vi "Dashboard Main.vi"() -> ()   [LabVIEW 2013]
uses:
  <vilib>/event_ctls.llb/eventvkey.ctl
  <vilib>/Rock Robotics/WPI/Dashboard/WPI_DashboardLogging Global.vi
  <vilib>/Utility/config.llb/Write Key (String).vi
  <vilib>/Utility/config.llb/Write Key (I32).vi
  <vilib>/Utility/config.llb/NI_LVConfig.lvlib
panel:
  out "Image Message":string="Timeout in Camera Communications"
  in  "Rec Mode":enum32{"Stop", "Record", "Playback"}(radio)
  in  "Dashboard Tab":T1(tab)
  out "Maybe\nShoot?":bool
  out "DISTANCE":dbl
  in  "Camera Settings":T2={"Frame Rate"=30, "Compression"=30, "Size"=1} {"Frame Rate" scale=1.0..30.0; "Size" items=["640x480", "320x240", "160x120"]}
  out "MotorSliders R":cluster{"MotorSlide1":dbl, "MotorSlide2":dbl} {"MotorSlide2" scale=-1.0..1.0 scale format="%#_2e"; "MotorSlide1" scale=-1.0..1.0 scale format="%#_2e"}
  out "MotorChart R":cluster{"Numeric":dbl, "Numeric":dbl}(graph)
  out "MotorSliders L":T3 {"MotorSlide4 2" scale=0.0..14.0 scale format="%#_2e"; "MotorSlide2" scale=-1.0..1.0 scale format="%#_2e"; "MotorSlide1" scale=-1.0..1.0 scale format="%#_2e"}
  out "MotorChart L":T4(graph)
  out "JS1 Z":dbl(slide) scale=-1.0..1.0 scale format="%#_2e"
  out "Joystick 1":cluster{"X":dbl, "Y":dbl}[](graph)
  out "JS Buttons 1":T5
  out "Twist-Handle":dbl(slide) scale=-1.0..1.0 scale format="%#_2e"
  out "Joystick 2":cluster{"X":dbl, "Y":dbl}[](graph)
  out "JS Buttons 2":T5
  out "Mode":T6(ring)=enum."Auto Disabled"
  out "Camera IP":string
  in  "DB Camera Config":bool
  out "fps":dbl format="%#.1g"
  out "Mbps":dbl format="%#.1g"
  out "Mbps 2":bool
  out "LED 1":bool
  out "Gamepad JS 1":cluster{"X":dbl, "Y":dbl}[](graph)
  out "Gamepad Buttons":T5
  out "GP1 Triggers":dbl(slide) scale=-1.0..1.0 scale format="%#_2e"
  out "Gamepad JS 2":cluster{"X":dbl, "Y":dbl}[](graph)
  out "R-JS Throttle":dbl(slide) scale=-1.0..1.0 scale format="%#_2e"
  in  "Stop Button":bool
  in  "Control Mode":u16(ring) items=["Gamepad", "Joystick"]
  out "Limit Switches":T7
  in  "Checkbox 2":bool
  in  "Checkbox 1":bool
  in  "Test Slider":dbl(slide) scale=0.0..100.0 scale format="%#_3g"
  in  "On/Off":bool caption="Solenoid"
  in  "Test Name":u16(ring) items=["Select the test to run...", "Example Test", "-------------------------------", "List of tests is built in robot code.", "Replace with your own automated tests."]
  in  "Test Tree":string(tree)
  in  "Motor":cluster{"Value":dbl, "Enable":bool} {"Value" scale=-1.0..1.0 scale format="%#_3g"}
  out "Progress":T8 {"Test Progress" scale=0.0..100.0}
  in  "Rev/Fwd":cluster{"Forward":bool, "Reverse":bool}
  in  "Test Ring":u16(ring) items=["Auto", "Fixed indoor", "Fixed outdoor 1", "Fixed outdoor 2", "Fixed fluorescent 1", "Fixed fluorescent 2", "Hold current"]
  in  "Listbox":i32(listbox)
  out "Tree":string(tree)
  out "Camera Image":T9(plugin-control)
  in  "Enable":bool
  # "Gamepad 1"
  # "Auxiliary Joystick"
  # "Rotational Joystick"
  # "Left"
  # "Front"
  # "Right"
  # "Battery"
  # "This tab is a great place for autonomous settings and validation.\nCustomize by placing controls and indicators here and name to\nmatch Dashboard Variables on robot."
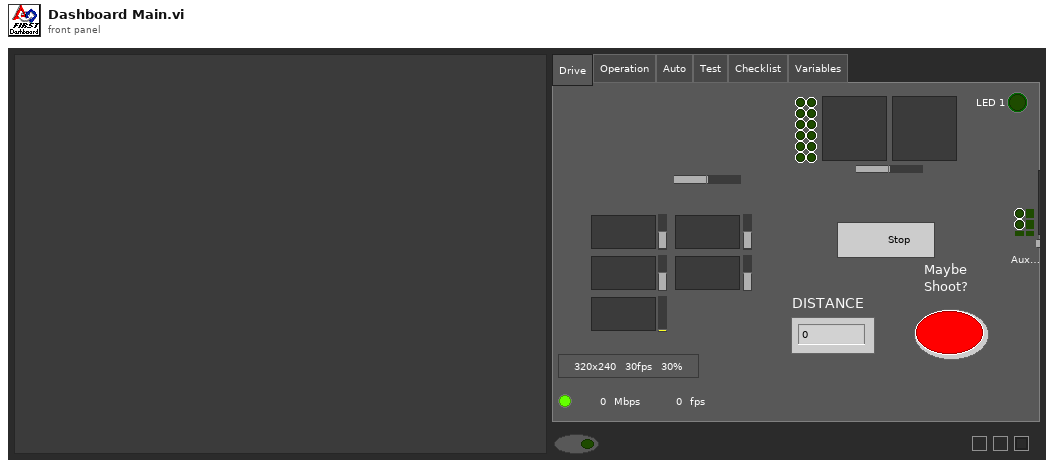
[diagram p1: front panel]
types:
  T1 = enum32{"Drive", "Operation", "Auto", "Test", "Checklist", "Variables"}
  T2 = cluster{"Frame Rate":i32, "Compression":i32, "Size":u16}
  T3 = cluster{"MotorSlide1":dbl, "MotorSlide2":dbl, "MotorSlide4 2":dbl}
  T4 = cluster{"Numeric":dbl, "Numeric":dbl, "Battery":sgl}
  T5 = cluster{bool, bool, bool, bool, bool, bool, bool, bool, bool, bool, bool, bool}
  T6 = enum8{"Tele-Op Disabled", "Tele-Op Enabled", "Auto Disabled", "Auto Enabled", "Test Disabled", "Test Enabled", ""}
  T7 = cluster{"PU Top":bool, "PU Bottom":bool, "Shoot Bottom":bool, "Shoot Top":bool}
  T8 = cluster{"Test Progress":u8, "Test Progress Text":string}
  T9 = typedef "IMAQ Image.ctl" = refnum<image>
  T10 = typedef "Image Type" = u32
  T11 = cluster{"Digital Inputs":bool[], "Digital Outputs":bool[]}
  T12 = cluster{"Competition mode":bool, "Robot Link":bool, "Autonomous":bool, "Enabled":bool, "E-Stop":bool, "Simulated":bool, "TestMode":bool, "Docked Window":bool}
  T13 = cluster{"Boolean Array[0]":bool, "Boolean Array[1]":bool, "Boolean Array[2]":bool, "Boolean Array[3]":bool, "Boolean Array[4]":bool, "Boolean Array[5]":bool, "Boolean Array[6]":bool, "Boolean Array[7]":bool, "Boolean Array[8]":bool, "Boolean Array[9]":bool, "Boolean Array[10]":bool, "Boolean Array[11]":bool}
  T14 = cluster{"Boolean Array[0]":bool, "Boolean Array[1]":bool, "Boolean Array[2]":bool, "Boolean Array[3]":bool}
  T15 = typedef "NI_LVConfig.lvlib/Config Data RefNum.ctl" = refnum<k1>
  T16 = typedef "eventvkey.ctl" = enum16{"ASCII", "Enter", "Return", "Shift", "Ctrl", "Alt", "Cmd", "Opt", "Caps", "NumLock", "Clear", "Break", "Up", "Down", "Left", "Right", "Insert", "Delete", "Home", "End", "PageUp", "PageDown", "Escape", "Help", "Pause", "ScrollLock", "F1", "F2", "F3", "F4", "F5", "F6", "F7", "F8", "F9", "F10", "F11", "F12", "F13", "F14", "F15", "F16", "F17", "F18", "F19", "F20", "F21", "F22", "F23", "F24", "Play", "VolumeUp", "VolumeDown", "Mute", "Two Byte Char"}
  T17 = cluster{"Image Size":bool, "Image Type":bool, "Pixel Value":bool, "ROI Information":bool, "Zoom Factor":bool}
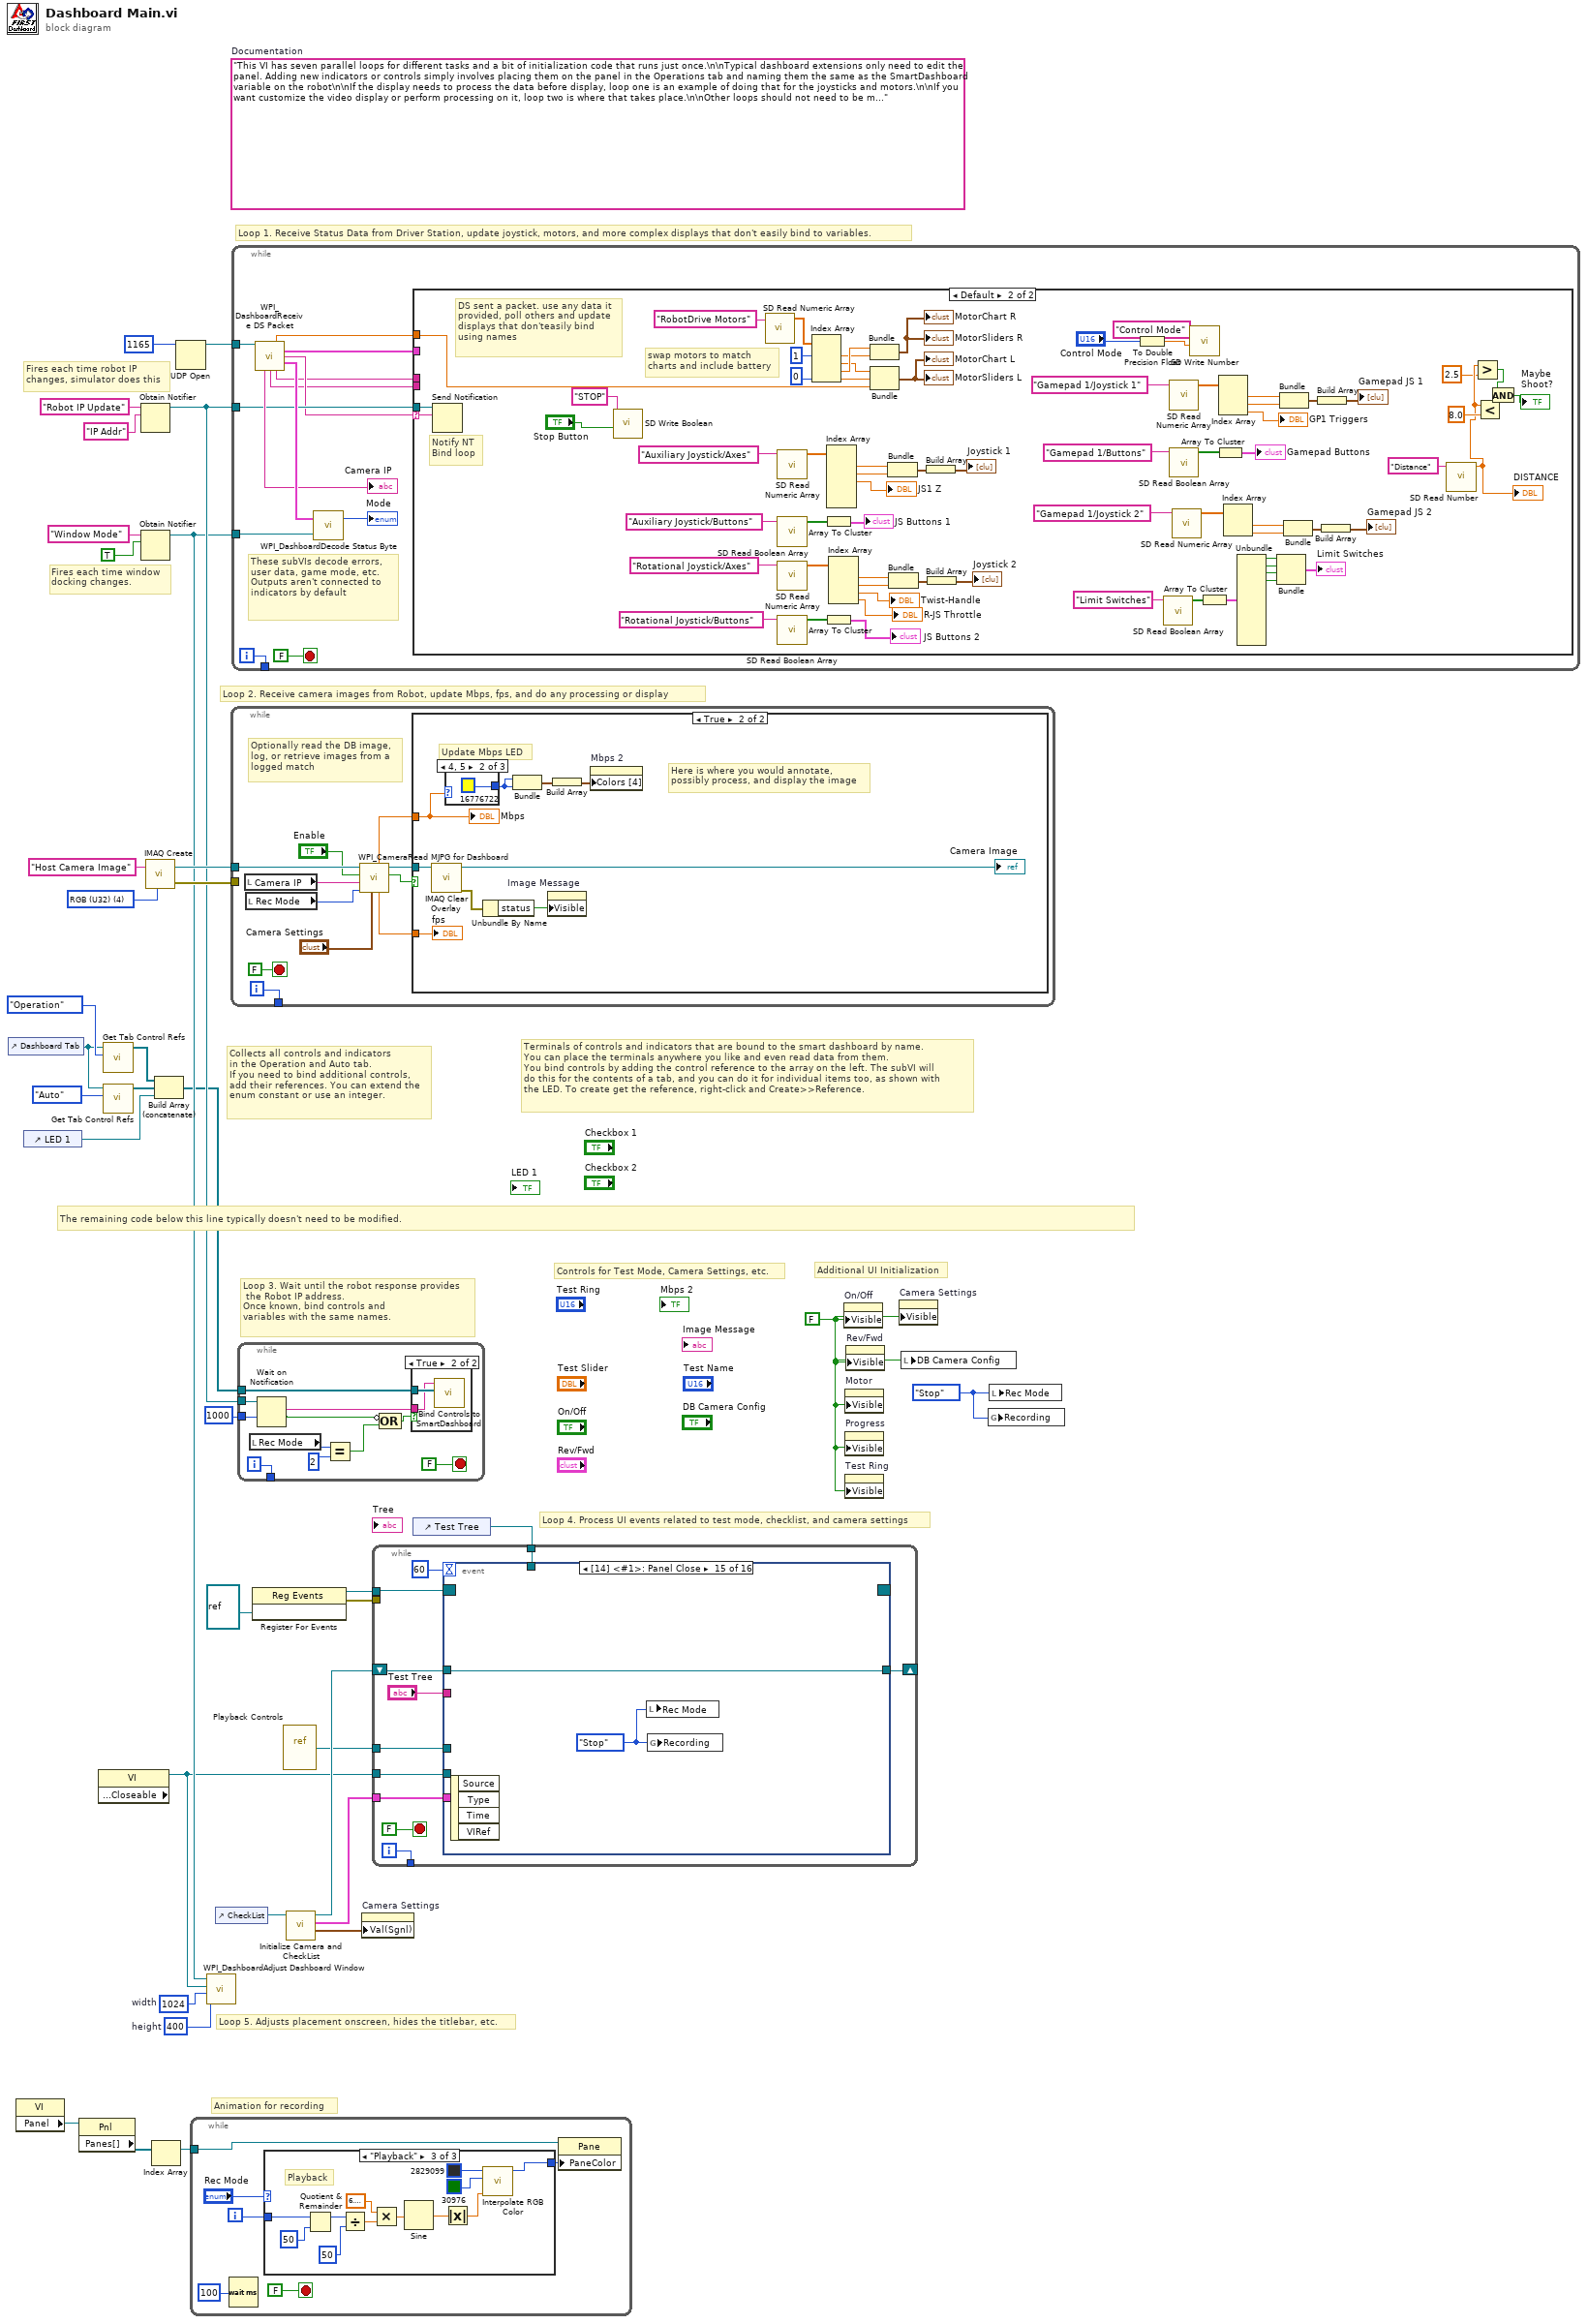
[diagram p0: block diagram]
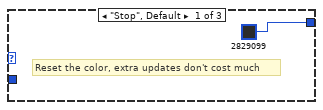
[diagram p2: hidden frame]
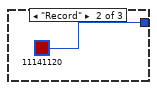
[diagram p3: hidden frame]
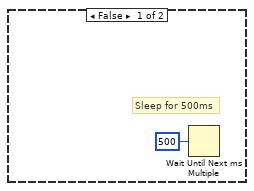
[diagram p5: hidden frame]
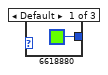
[diagram p6: hidden frame]
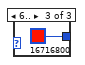
[diagram p7: hidden frame]
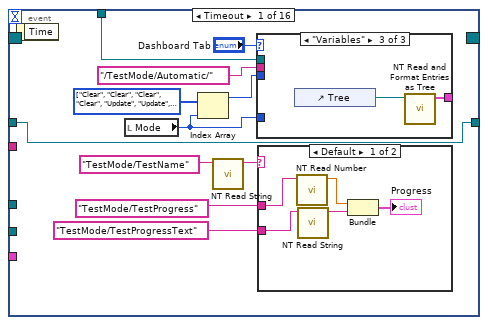
[diagram p8: hidden frame]
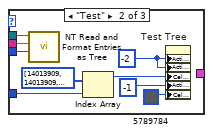
[diagram p10: hidden frame]
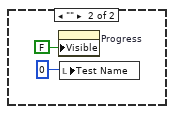
[diagram p11: hidden frame]
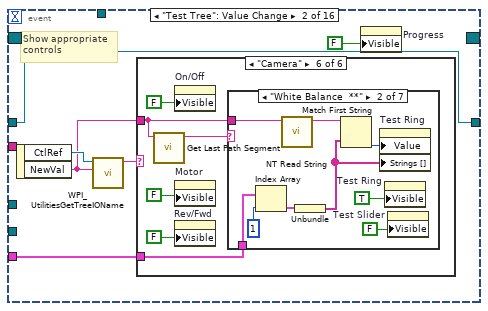
[diagram p12: hidden frame]
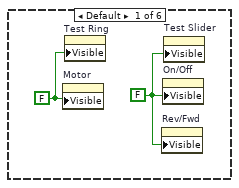
[diagram p13: hidden frame]
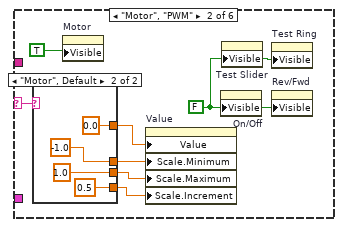
[diagram p14: hidden frame]
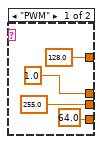
[diagram p15: hidden frame]
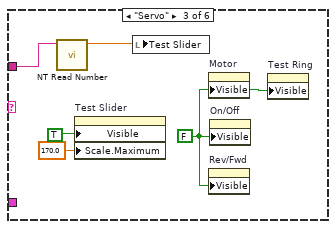
[diagram p16: hidden frame]
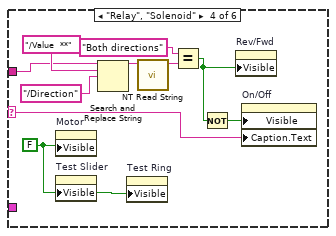
[diagram p17: hidden frame]
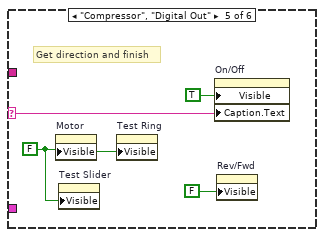
[diagram p18: hidden frame]
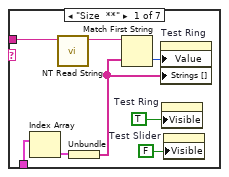
[diagram p19: hidden frame]
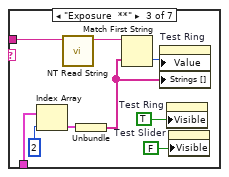
[diagram p20: hidden frame]
diagram:
  w8 = enum32{"Stop", "Record", "Playback"}."Stop" ("Rec Mode")
  w11 = 400  # height
  w12 = 1024  # width
  w25 = FALSE ("Visible")
  (unwired) "This VI has seven parallel loops for different tasks and a bit of initialization code that runs just once.\n\nTypical dashboard extensions only need to edit the panel. Adding new indicators or controls simply involves placing them on the panel in the Operations tab and naming them the same as the SmartDashboard variable on the robot\n\nIf the display needs to process the data before display, loop one is an example of doing that for the joysticks and motors.\n\nIf you want customize the video display or perform processing on it, loop two is where that takes place.\n\nOther loops should not need to be modified. They are pretty standard, and document the task they perform."  # Documentation
  w35 = T10 4 items=["Grayscale (U8)", "Grayscale (I16)", "Grayscale (SGL)", "Complex (CSG)", "RGB (U32)", "HSL (U32)", "RGB (U64)"] ("Image Type")
  # "Controls for Test Mode, Camera Settings, etc."
  # "Additional UI Initialization"
  # "Animation for recording"
  # "Fires each time robot IP\nchanges, simulator does this"
  # "Fires each time window\ndocking changes."
  # "Collects all controls and indicators\nin the Operation and Auto tab.\nIf you need to bind additional controls,\nadd their references. You can extend the\nenum constant or use an integer."
  # "The remaining code below this line typically doesn't need to be modified."
  # "Loop 4. Process UI events related to test mode, checklist, and camera settings"
  # "Terminals of controls and indicators that are bound to the smart dashboard by name.\nYou can place the terminals anywhere you like and even read data from them.\nYou bind controls by adding the control reference to the array on the left. The subVI will\ndo this for the contents of a tab, and you can do it for individual items too, as shown with\nthe LED. To create get the reference, right-click and Create>>Reference."
  # "Loop 3. Wait until the robot response provides\n the Robot IP address.\nOnce known, bind controls and\nvariables with the same names."
  # "Loop 5. Adjusts placement onscreen, hides the titlebar, etc."
  # "Loop 1. Receive Status Data from Driver Station, update joystick, motors, and more complex displays that don't easily bind to variables."
  # "Loop 2. Receive camera images from Robot, update Mbps, fps, and do any processing or display"
  n1 = control-ref of="Dashboard Tab"() -> (w6:refnum<vi>)
  n2 = property class="VI"() -> ("Panel"=w19:refnum<vi>)  [unwired: 2 in, 2 out]
  n3 = control-ref of="LED 1"() -> (w1:refnum<vi>)
  n4 = property class="Pnl"(reference=w19) -> ("Panes[]"=w20:refnum<vi>[])  [unwired: 1 in, 2 out]
  n5 = property class="VI" props=["Front Panel.Closeable"]() -> (reference out=w7:refnum<vi>)  [unwired: 2 in, 2 out]
  n6 = call <vilib>:"Get Tab Control Refs.vi"("Page Index"=T1."Operation" ("Dashboard Tab"), "TabControl in"=w6) -> ("ControlsOnPage"=w4:refnum<vi>[])  [unwired: 9 in]
  n7 = call <vilib>:"Get Tab Control Refs.vi"("Page Index"=T1."Auto" ("Dashboard Tab"), "TabControl in"=w6) -> ("ControlsOnPage"=w5:refnum<vi>[])  [unwired: 9 in]
  n8 = Obtain Notifier(name (unnamed)="Robot IP Update", notification data type="IP Addr" ("name (unnamed)")) -> (notifier out=w29:refnum<notifier>)  [unwired: 2 in, 2 out]
  n9 = Obtain Notifier(name (unnamed)="Window Mode", notification data type=TRUE) -> (notifier out=w10:refnum<notifier>)  [unwired: 2 in, 2 out]
  n10 = call "IMAQ Create"("Image Name"="Host Camera Image", "Image Type"=w35) -> ("New Image"=w33:T9, "error out"=w32:errorcluster)  [unwired: 2 in, 1 out]
  n11 = Index Array(array=w20) -> (element=w18:refnum<vi>)  [unwired: 1 in]
  n12 = Build Array (concatenate)(w4, w5, w1) -> (w3:refnum<vi>[])
  n13 = UDP Open(11:u16 1165 ("port")) -> (port=w36:refnum<k16>)  [unwired: 2 in, 4 out]
  n14 = while {
    tunnel: w18 -> [w39]
    i -> [w42]
    stop <- FALSE stop-if-true
    n15 = Wait (ms)(milliseconds to wait=u32 100) -> ()  [unwired: 1 out]
    n16 = case shown="\"Playback\"" "Rec Mode" {
      tunnel: w42 -> [_ _ w57]
      tunnel: [u32 2829099 ("Base Color") u32 11141120 ("Target Color") w46] -> w38
      frame "Stop", Default {
        # "Reset the color, extra updates don't cost much"
      }
      frame "Record" {
      }
      frame "Playback" {
        # "Playback"
        n17 = Quotient & Remainder(x=w57, y=u32 50 ("milliseconds to wait")) -> (x-y*floor(x/y)=w53:u32)  [unwired: 1 out]
        n18 = Divide(x=w53, y=u32 50 ("milliseconds to wait")) -> (x/y=w50:dbl)
        n19 = Multiply(x=6.283185307179586, y=w50) -> (x*y=w55:dbl)
        n20 = Sine(x=w55) -> (sin(x)=w54:dbl)
        n21 = Absolute Value(x=w54) -> (abs(x)=w47:dbl)
        n22 = call "Interpolate RGB Color.vi"("Proportion"=w47, "Target Color"=u32 30976, "Base Color"=u32 2829099) -> ("Result Color"=w46:u32)  [unwired: 8 in]
      }
    }
    n23 = property class="Pane"(reference=w39, "PaneColor"=w38) -> ()  [unwired: 1 in, 2 out]
  }
  n24 = call <vilib>:"WPI_DashboardAdjust Dashboard Window.vi"("height"=w11, "width"=w12, "reference in"=w7, "Notifier in"=w10) -> ()  [unwired: 8 in]
  n25 = control-ref of="CheckList"() -> (w9:refnum<vi>)
  n26 = while {
    tunnel: w33 -> [w66]
    tunnel: w32 -> [_]
    tunnel: [w67] -> _
    i -> [w67]
    stop <- FALSE stop-if-true
    # "Optionally read the DB image,\nlog, or retrieve images from a\nlogged match"
    n27 = local read "Camera IP"() -> (w59:string)
    n28 = local read "Rec Mode"() -> (w58:enum32{"Stop", "Record", "Playback"})
    n29 = call <vilib>:"WPI_CameraRead MJPG for Dashboard.vi"("Camera Settings"="Camera Settings", "Rec Mode"=w58, "Camera IP"=w59, "Enable"="Enable", "Refnum in"=w66) -> ("Active"=w63:bool, "Refnum out"=w65:T9, "FPS"=w62:dbl, "Bandwidth (Mbps)"=w61:dbl)  [unwired: 3 in]
    n30 = case shown="True" w63 {
      tunnel: w65 -> [_ w73]
      tunnel: w61 -> [_ w72]
      tunnel: w62 -> [_ w70]
      frame False {
        # "Sleep for 500ms"
        n31 = Wait Until Next ms Multiple(millisecond multiple=u32 500) -> ()  [unwired: 1 out]
      }
      frame True {
        # "Here is where you would annotate,\npossibly process, and display the image"
        # "Update Mbps LED"
        n32 = call "IMAQ Clear Overlay"("Image"=w73) -> ("error out"=w77:errorcluster, "Image Out"=→"Camera Image":T9)  [unwired: 2 in, 7 out]
        n33 = case shown="4, 5" w72 {
          tunnel: [u32 6618880 ("Color Box") u32 16776722 ("Color Box") u32 16716800 ("Color Box")] -> w74
          frame Default {
          }
          frame 4, 5 {
          }
          frame 6.. {
          }
        }
        n34 = Unbundle By Name(w77) -> ("status"=w78:bool)
        n35 = Bundle("Color Box"=w74, "Color Box"=w74) -> (w76:cluster{"Color Box":u32, "Color Box":u32})  [unwired: 1 out]
        n36 = property on="Image Message" class="Str"("Visible"=w78) -> ()  [unwired: 2 in, 2 out]
        n37 = Build Array(w76) -> (w75:cluster{"Color Box":u32, "Color Box":u32}[])
        n38 = property on="Mbps 2" class="Bool (strict)"("Colors [4]"=w75) -> ()  [unwired: 2 in, 2 out]
        "Mbps" <- w72
        "fps" <- w70
      }
    }
  }
  n39 = while {
    tunnel: w36 -> [w92]
    tunnel: w29 -> [w87]
    tunnel: w10 -> [w91]
    tunnel: [w88] -> _
    i -> [w88]
    stop <- FALSE stop-if-true
    # "These subVIs decode errors, user data, game mode, etc.\nOutputs aren't connected to indicators by default"
    n40 = call <vilib>:"WPI_DashboardReceive DS Packet.vi"("Recv Socket"=w92) -> ("Battery"=w82:sgl, "Driver Station"=w83:T11, "Robot IP Address"=w86:string, "Status"=w93:T12, "Camera IP Address"=→"Camera IP":string, "Low Priority User Data"=w85:string, "High Priority User Data"=w84:string)  [unwired: 1 in, 7 out]
    n41 = call <vilib>:"WPI_DashboardDecode Status Byte.vi"("Window Mode Notifier"=w91, "Status"=w93) -> ("Mode"=→"Mode":T6)  [unwired: 1 out]
    n42 = case shown="Default" w86 {
      selector: w86 -> [_ w142]
      tunnel: w87 -> [_ w143]
      tunnel: w85 -> [_ _]
      tunnel: w84 -> [_ _]
      tunnel: w83 -> [_ _]
      tunnel: w82 -> [_ w141]
      frame "0.0.0.0" {
        # "DS not sending packets, or no robot exists yet.\nDon't poll the variables"
      }
      frame Default {
        # "Notify NT\nBind loop"
        # "DS sent a packet. use any data it\nprovided, poll others and update\ndisplays that don'teasily bind\nusing names"
        # "swap motors to match\ncharts and include battery"
        n43 = Send Notification(notification=w142, notifier=w143) -> ()  [unwired: 1 in, 2 out]
        n44 = call <vilib>:"SD Write Boolean.vi"("Boolean"="Stop Button", "Name"="STOP") -> ()  [unwired: 8 in, 2 out]
        n45 = call <vilib>:"SD Read Numeric Array.vi"("Name"="RobotDrive Motors") -> ("Numeric Array"=w140:dbl[])  [unwired: 8 in, 2 out]
        n46 = call <vilib>:"SD Read Numeric Array.vi"("Name"="Auxiliary Joystick/Axes") -> ("Numeric Array"=w159:dbl[])  [unwired: 8 in, 2 out]
        n47 = call <vilib>:"SD Read Boolean Array.vi"("Name"="Auxiliary Joystick/Buttons") -> ("Boolean Array"=w161:bool[])  [unwired: 8 in, 2 out]
        n48 = call <vilib>:"SD Read Numeric Array.vi"("Name"="Rotational Joystick/Axes") -> ("Numeric Array"=w153:dbl[])  [unwired: 8 in, 2 out]
        n49 = call <vilib>:"SD Read Boolean Array.vi"("Name"="Rotational Joystick/Buttons") -> ("Boolean Array"=w152:bool[])  [unwired: 8 in, 2 out]
        n50 = Index Array(array=w140, index #1=1, index #4=0) -> (element #1=w136:dbl, element #2=w135:dbl, element #3=w137:dbl, element #4=w132:dbl)  [unwired: 2 in]
        n51 = Array To Cluster(array=w161) -> (cluster=→"JS Buttons 1":T13)
        n52 = Array To Cluster(array=w152) -> (cluster=→"JS Buttons 2":T13)
        n53 = Index Array(array=w159) -> (element #1=w156:dbl, element #2=w157:dbl, element #3=→"JS1 Z":dbl)  [unwired: 6 in, 3 out]
        n54 = Index Array(array=w153) -> (element #1=w148:dbl, element #2=w147:dbl, element #3=→"Twist-Handle":dbl, element #4=→"R-JS Throttle":dbl)  [unwired: 4 in]
        n55 = Bundle("Numeric"=w137, "Numeric"=w136) -> (→"MotorChart R" →"MotorSliders R":cluster{"Numeric":dbl, "Numeric":dbl})  [unwired: 1 in]
        n56 = Bundle("Numeric"=w135, "Numeric"=w132, "Battery"=w141) -> (→"MotorChart L" →"MotorSliders L":T4)  [unwired: 1 in]
        n57 = Bundle("Numeric"=w156, "Numeric"=w157) -> (w155:cluster{"Numeric":dbl, "Numeric":dbl})  [unwired: 1 in]
        n58 = Bundle("Numeric"=w148, "Numeric"=w147) -> (w149:cluster{"Numeric":dbl, "Numeric":dbl})  [unwired: 1 in]
        n59 = Build Array(w155) -> (→"Joystick 1":cluster{"Numeric":dbl, "Numeric":dbl}[])
        n60 = Build Array(w149) -> (→"Joystick 2":cluster{"Numeric":dbl, "Numeric":dbl}[])
        n61 = To Double Precision Float(number="Control Mode") -> (double precision float=w105:dbl)
        n62 = call <vilib>:"SD Read Boolean Array.vi"("Name"="Limit Switches") -> ("Boolean Array"=w114:bool[])  [unwired: 8 in, 2 out]
        n63 = call <vilib>:"SD Read Numeric Array.vi"("Name"="Gamepad 1/Joystick 1") -> ("Numeric Array"=w127:dbl[])  [unwired: 8 in, 2 out]
        n64 = call <vilib>:"SD Read Boolean Array.vi"("Name"="Gamepad 1/Buttons") -> ("Boolean Array"=w129:bool[])  [unwired: 8 in, 2 out]
        n65 = call <vilib>:"SD Read Numeric Array.vi"("Name"="Gamepad 1/Joystick 2") -> ("Numeric Array"=w121:dbl[])  [unwired: 8 in, 2 out]
        n66 = call <vilib>:"SD Write Number.vi"("Numeric"=w105, "Name"="Control Mode") -> ()  [unwired: 8 in, 2 out]
        n67 = Array To Cluster(array=w114) -> (cluster=w113:T13)
        n68 = Array To Cluster(array=w129) -> (cluster=→"Gamepad Buttons":T13)
        n69 = Index Array(array=w127) -> (element #1=w124:dbl, element #2=w125:dbl, element #3=→"GP1 Triggers":dbl)  [unwired: 3 in]
        n70 = Index Array(array=w121) -> (element #1=w118:dbl, element #2=w117:dbl)  [unwired: 2 in]
        n71 = Unbundle(w113) -> ("Boolean Array[0]"=w112:bool, "Boolean Array[1]"=w111:bool, "Boolean Array[2]"=w110:bool, "Boolean Array[3]"=w109:bool)  [unwired: 8 out]
        n72 = Bundle("Boolean Array[0]"=w112, "Boolean Array[1]"=w111, "Boolean Array[2]"=w110, "Boolean Array[3]"=w109) -> (→"Limit Switches":T14)  [unwired: 1 in]
        n73 = Bundle("Numeric"=w124, "Numeric"=w125) -> (w123:cluster{"Numeric":dbl, "Numeric":dbl})  [unwired: 1 in]
        n74 = Bundle("Numeric"=w118, "Numeric"=w117) -> (w119:cluster{"Numeric":dbl, "Numeric":dbl})  [unwired: 1 in]
        n75 = Build Array(w123) -> (→"Gamepad JS 1":cluster{"Numeric":dbl, "Numeric":dbl}[])
        n76 = Build Array(w119) -> (→"Gamepad JS 2":cluster{"Numeric":dbl, "Numeric":dbl}[])
        n77 = call <vilib>:"SD Read Number.vi"("Name"="Distance") -> ("Numeric"=w99:dbl)  [unwired: 8 in, 2 out]
        "DISTANCE" <- w99
        n78 = Greater?(x=w99, y=2.5) -> (0:w97:bool)
        n79 = Less?(x=w99, y=8.0) -> (x < y?=w96:bool)
        n80 = And(x=w97, y=w96) -> (x .and. y?=→"Maybe\nShoot?":bool)
      }
    }
  }
  n81 = while {
    tunnel: w3 -> [w175]
    tunnel: w29 -> [w173]
    tunnel: [w171] -> _
    tunnel: u32 1000 ("milliseconds to wait") -> [w170]
    i -> [w171]
    stop <- FALSE stop-if-true
    n82 = local read "Rec Mode"() -> (w166:enum32{"Stop", "Record", "Playback"})
    n83 = Wait on Notification(notifier=w173, timeout in ms (-1)=w170) -> (notification=w172:string, timed out?=w168:bool)  [unwired: 2 in, 2 out]
    n84 = Equal?(x=w166, y=u16 2 ("Rec Mode")) -> (x = y?=w167:bool)
    n85 = Compound Arithmetic op=OR(invert w168, w167) -> (w169:bool)
    n86 = case shown="True" w169 {
      tunnel: w175 -> [_ w177]
      tunnel: w172 -> [_ w176]
      frame False {
      }
      frame True {
        n87 = call <vilib>:"Bind Controls to SmartDashboard.vi"("Bound Control Refs"=w177, "Server IP Address"=w176) -> ()  [unwired: 10 in]
      }
    }
  }
  n88 = register-events(refnum<vi> refnum) -> (reference out=w16:refnum<event-registration>, error out=w15:errorcluster)  [unwired: 2 in]
  n89 = vi-ref "Playback Controls.vi"() -> (w17:refnum<vi>)
  n90 = call "Initialize Camera and CheckList.vi"("ListBox in"=w9) -> ("Cluster"=w23:cluster{"value":i32, "value":i32, "index":i32}, "Array"=w24:cluster{string[]}[], "File Refnum"=w22:T15)  [unwired: 8 in]
  n91 = property on="Camera Settings" class="Clust (strict)"("Val(Sgnl)"=w23) -> ()  [unwired: 2 in, 2 out]
  n92 = control-ref of="Test Tree"() -> (w21:refnum<vi>)
  n93 = while {
    tunnel: w24 -> [w185]
    shift-right: [w184] -> _
    shift-left: w22 -> [w183]
    tunnel: [w182] -> _
    tunnel: w21 -> [w181]
    tunnel: w17 -> [w180]
    tunnel: w16 -> [w179]
    tunnel: w15 -> [_]
    tunnel: w7 -> [w178]
    i -> [w182]
    stop <- FALSE stop-if-true
    n94 = event shown="[14] <#1>: Panel Close" {
      selector: w179 -> [_ _ _ _ _ _ _ _ _ _ _ _ _ _ _ _]
      dyn-events: [_ _ _ _ _ _ _ _ _ _ _ _ _ w423 _ _] -> _
      timeout: u32 60 ("milliseconds to wait") -> [_ _ _ _ _ _ _ _ _ _ _ _ _ _ _ _]
      tunnel: w181 -> [w195 _ _ _ _ _ _ _ _ _ _ _ _ _ _ _]
      tunnel: "Test Tree" -> [_ _ _ _ _ _ _ _ w392 w400 w402 w406 w414 _ _ _]
      tunnel: w185 -> [_ w219 _ _ _ _ w356 w386 _ _ _ _ _ _ _ _]
      tunnel: [w189 w218 w317 w322 w330 w342 w355 w379 w391 w398 w401 w405 w413 w425 w439 w440] -> w184
      tunnel: w183 -> [w189 w218 w317 w322 w330 w342 w354 w379 w391 w398 w401 w405 w413 w425 w439 w440]
      tunnel: w180 -> [_ _ _ _ _ _ _ _ _ _ _ _ _ w426 _ w443]
      tunnel: w178 -> [_ _ _ _ _ _ _ _ _ _ _ _ _ w421 _ _]
      event Timeout {
        w194 = enum16{"Update", "Clear"}[] [enum."Clear", enum."Clear", enum."Clear", enum."Clear", enum."Update", enum."Update", enum."Clear"] items=["Update", "Clear"]
        n95 = event-data() -> ()  [unwired: 1 in, 1 out]
        n96 = local read "Mode"() -> (w192:T6)
        n97 = Index Array(array=w194, index=w192) -> (element=w193:enum16{"Update", "Clear"})
        n98 = call <vilib>:"NT Read String.vi"("Name"="TestMode/TestName") -> ("String"=w198:string)  [unwired: 9 in, 1 out]
        n99 = case shown="\"Variables\"" "Dashboard Tab" {
          tunnel: w195 -> [_ w208 _]
          tunnel: "/TestMode/Automatic/" ("Name Pattern") -> [_ w207 _]
          tunnel: w193 -> [_ w206 _]
          tunnel: w192 -> [_ w204 _]
          tunnel: [_ _ w210] -> _
          frame "Operation", Default {
          }
          frame "Test" {
            w203 = -2 ("Active Item:Row Number")
            n100 = call <vilib>:"NT Read and Format Entries as Tree.vi"("Operation"=w206, "Name Pattern"=w207, "Tree Refnum"=w208) -> ()  [unwired: 7 in, 2 out]
            n101 = Index Array(array=u32[] [14013909, 14013909, 14013909, 14013909, 14013909, 16777215, 14013909], index=w204) -> (element=w202:u32)
            n102 = property on="Test Tree" class="Tree (strict)"("Active Item Row Number"=w203, "ActiveColNum"=w203, "CellBG"=w202, "Active Item Row Number"=-1 ("Active Item:Row Number"), "CellBG"=u32 5789784 ("Color Box")) -> ()  [unwired: 2 in, 2 out]
          }
          frame "Variables" {
            n103 = control-ref of="Tree"() -> (w209:refnum<vi>)
            n104 = call <vilib>:"NT Read and Format Entries as Tree.vi"("Tree Refnum"=w209) -> ("Formatted Strings"=w210:cluster{"Name":string, "Value":string}[])  [unwired: 9 in, 1 out]
          }
        }
        n105 = case shown="Default" w198 {
          tunnel: "TestMode/TestProgress" ("Name") -> [w212 _]
          tunnel: "TestMode/TestProgressText" ("Name") -> [w211 _]
          frame Default {
            n106 = call <vilib>:"NT Read Number.vi"("Name"=w212) -> ("Numeric"=w213:dbl)  [unwired: 9 in, 1 out]
            n107 = call <vilib>:"NT Read String.vi"("Name"=w211) -> ("String"=w214:string)  [unwired: 9 in, 1 out]
            n108 = Bundle("Numeric"=w213, "String"=w214) -> (→"Progress":cluster{"Numeric":dbl, "String":string})  [unwired: 1 in]
          }
          frame "" {
            n109 = property on="Progress" class="Clust (strict)"("Visible"=FALSE) -> ()  [unwired: 2 in, 2 out]
            n110 = local write "Test Name"(u16 0) -> ()
          }
        }
      }
      event "Test Tree": Value Change {
        # "Show appropriate\ncontrols"
        n111 = event-data() -> ("CtlRef"=w222:refnum<vi>, "NewVal"=w220:string)  [unwired: 1 in]
        n112 = call <vilib>:"WPI_UtilitiesGetTreeIOName.vi"("NewVal"=w220, "TreeControl in"=w222) -> ("I/O Name"=w223:string)  [unwired: 9 in]
        n113 = case shown="\"Camera\"" w223 {
          selector: w223 -> [_ w230 _ w248 w257 _]
          tunnel: w220 -> [_ _ w245 w247 _ w264]
          tunnel: w219 -> [_ _ _ _ _ w263]
          frame Default {
            w225 = FALSE ("Visible")
            w224 = FALSE ("Visible")
            n114 = property on="Motor" class="Clust (strict)"("Visible"=w224) -> ()  [unwired: 2 in, 2 out]
            n115 = property on="Test Ring" class="Ring (strict)"("Visible"=w224) -> ()  [unwired: 2 in, 2 out]
            n116 = property on="Rev/Fwd" class="Clust (strict)"("Visible"=w225) -> ()  [unwired: 2 in, 2 out]
            n117 = property on="On/Off" class="Bool (strict)"("Visible"=w225) -> ()  [unwired: 2 in, 2 out]
            n118 = property on="Test Slider" class="Slide (strict)"("Visible"=w225) -> ()  [unwired: 2 in, 2 out]
          }
          frame "Motor", "PWM" {
            w231 = FALSE ("Visible")
            n119 = case shown="\"Motor\", Default" w230 {
              tunnel: [1.0 ("Value") -1.0 ("Value")] -> w229
              tunnel: [255.0 ("Value") 1.0 ("Value")] -> w228
              tunnel: [128.0 ("Value") 0.0 ("Value")] -> w227
              tunnel: [64.0 ("Value") 0.5 ("Value")] -> w226
              frame "PWM" {
              }
              frame "Motor", Default {
              }
            }
            n120 = property on="Motor" class="Clust (strict)"("Visible"=TRUE) -> ()  [unwired: 2 in, 2 out]
            n121 = property on="Value" class="Slide (strict)"("Value"=w227, "Scale.Minimum"=w229, "Scale.Maximum"=w228, "Scale.Increment"=w226) -> ()  [unwired: 2 in, 2 out]
            n122 = property on="On/Off" class="Bool (strict)"("Visible"=w231) -> ()  [unwired: 2 in, 2 out]
            n123 = property on="Test Slider" class="Slide (strict)"("Visible"=w231) -> ()  [unwired: 2 in, 2 out]
            n124 = property on="Test Ring" class="Ring (strict)"("Visible"=w231) -> ()  [unwired: 2 in, 2 out]
            n125 = property on="Rev/Fwd" class="Clust (strict)"("Visible"=w231) -> ()  [unwired: 2 in, 2 out]
          }
          frame "Servo" {
            w243 = FALSE ("Visible")
            n126 = call <vilib>:"NT Read Number.vi"("Name"=w245) -> ("Numeric"=w244:dbl)  [unwired: 9 in, 1 out]
            n127 = property on="Test Slider" class="Slide (strict)"("Visible"=TRUE, "Scale.Maximum"=170.0 ("Scale.Range:Maximum")) -> ()  [unwired: 2 in, 2 out]
            n128 = local write "Test Slider"(w244) -> ()
            n129 = property on="Motor" class="Clust (strict)"("Visible"=w243) -> ()  [unwired: 2 in, 2 out]
            n130 = property on="Rev/Fwd" class="Clust (strict)"("Visible"=w243) -> ()  [unwired: 2 in, 2 out]
            n131 = property on="On/Off" class="Bool (strict)"("Visible"=w243) -> ()  [unwired: 2 in, 2 out]
            n132 = property on="Test Ring" class="Ring (strict)"("Visible"=w243) -> ()  [unwired: 2 in, 2 out]
          }
          frame "Relay", "Solenoid" {
            w246 = FALSE ("Visible")
            n133 = property on="Motor" class="Clust (strict)"("Visible"=w246) -> ()  [unwired: 2 in, 2 out]
            n134 = property on="Test Slider" class="Slide (strict)"("Visible"=w246) -> ()  [unwired: 2 in, 2 out]
            n135 = Search and Replace String(input string=w247, search string="/Value  **", replace string="/Direction") -> (result string=w253:string)  [unwired: 5 in, 3 out]
            n136 = property on="Test Ring" class="Ring (strict)"("Visible"=w246) -> ()  [unwired: 2 in, 2 out]
            n137 = call <vilib>:"NT Read String.vi"("Name"=w253) -> ("String"=w251:string)  [unwired: 9 in, 1 out]
            n138 = Equal?(x="Both directions", y=w251) -> (x = y?=w249:bool)
            n139 = Not(x=w249) -> (.not. x?=w250:bool)
            n140 = property on="Rev/Fwd" class="Clust (strict)"("Visible"=w249) -> ()  [unwired: 2 in, 2 out]
            n141 = property on="On/Off" class="Bool (strict)"("Visible"=w250, "Caption.Text"=w248) -> ()  [unwired: 2 in, 2 out]
          }
          frame "Compressor", "Digital Out" {
            w256 = FALSE ("Visible")
            # "Get direction and finish"
            n142 = property on="Motor" class="Clust (strict)"("Visible"=w256) -> ()  [unwired: 2 in, 2 out]
            n143 = property on="Test Slider" class="Slide (strict)"("Visible"=w256) -> ()  [unwired: 2 in, 2 out]
            n144 = property on="Test Ring" class="Ring (strict)"("Visible"=w256) -> ()  [unwired: 2 in, 2 out]
            n145 = property on="On/Off" class="Bool (strict)"("Visible"=TRUE, "Caption.Text"=w257) -> ()  [unwired: 2 in, 2 out]
            n146 = property on="Rev/Fwd" class="Clust (strict)"("Visible"=FALSE) -> ()  [unwired: 2 in, 2 out]
          }
          frame "Camera" {
            n147 = call <vilib>:"Get Last Path Segment.vi"("String in"=w264) -> ("String out"=w265:string)  [unwired: 10 in]
            n148 = property on="On/Off" class="Bool (strict)"("Visible"=FALSE) -> ()  [unwired: 2 in, 2 out]
            n149 = property on="Motor" class="Clust (strict)"("Visible"=FALSE) -> ()  [unwired: 2 in, 2 out]
            n150 = property on="Rev/Fwd" class="Clust (strict)"("Visible"=FALSE) -> ()  [unwired: 2 in, 2 out]
            n151 = case shown="\"White Balance  **\"" w265 {
              tunnel: w264 -> [w271 w280 w289 w298 w307 _ w313]
              tunnel: w263 -> [w269 w277 w286 w295 w304 _ _]
              frame "Size  **" {
                n152 = Index Array(array=w269) -> (element=w268:cluster{string[]})  [unwired: 1 in]
                n153 = call <vilib>:"NT Read String.vi"("Name"=w271) -> ("String"=w270:string)  [unwired: 9 in, 1 out]
                n154 = Unbundle(w268) -> (w266:string[])
                n155 = Match First String(2:w266, 3:w270) -> (0:w267:i32)  [unwired: 1 out]
                n156 = property on="Test Ring" class="Ring (strict)"("Value"=w267, "Strings []"=w266) -> ()  [unwired: 2 in, 2 out]
                n157 = property on="Test Ring" class="Ring (strict)"("Visible"=TRUE) -> ()  [unwired: 2 in, 2 out]
                n158 = property on="Test Slider" class="Slide (strict)"("Visible"=FALSE) -> ()  [unwired: 2 in, 2 out]
              }
              frame "White Balance  **" {
                n159 = Index Array(array=w277, index=1) -> (element=w278:cluster{string[]})
                n160 = call <vilib>:"NT Read String.vi"("Name"=w280) -> ("String"=w279:string)  [unwired: 9 in, 1 out]
                n161 = Unbundle(w278) -> (w275:string[])
                n162 = Match First String(2:w275, 3:w279) -> (0:w274:i32)  [unwired: 1 out]
                n163 = property on="Test Ring" class="Ring (strict)"("Value"=w274, "Strings []"=w275) -> ()  [unwired: 2 in, 2 out]
                n164 = property on="Test Ring" class="Ring (strict)"("Visible"=TRUE) -> ()  [unwired: 2 in, 2 out]
                n165 = property on="Test Slider" class="Slide (strict)"("Visible"=FALSE) -> ()  [unwired: 2 in, 2 out]
              }
              frame "Exposure  **" {
                n166 = Index Array(array=w286, index=2) -> (element=w287:cluster{string[]})
                n167 = call <vilib>:"NT Read String.vi"("Name"=w289) -> ("String"=w288:string)  [unwired: 9 in, 1 out]
                n168 = Unbundle(w287) -> (w283:string[])
                n169 = Match First String(2:w283, 3:w288) -> (0:w284:i32)  [unwired: 1 out]
                n170 = property on="Test Ring" class="Ring (strict)"("Value"=w284, "Strings []"=w283) -> ()  [unwired: 2 in, 2 out]
                n171 = property on="Test Ring" class="Ring (strict)"("Visible"=TRUE) -> ()  [unwired: 2 in, 2 out]
                n172 = property on="Test Slider" class="Slide (strict)"("Visible"=FALSE) -> ()  [unwired: 2 in, 2 out]
              }
              frame "Exposure Priority  **" {
                n173 = Index Array(array=w295, index=3) -> (element=w296:cluster{string[]})
                n174 = call <vilib>:"NT Read String.vi"("Name"=w298) -> ("String"=w297:string)  [unwired: 9 in, 1 out]
                n175 = Unbundle(w296) -> (w292:string[])
                n176 = Match First String(2:w292, 3:w297) -> (0:w293:i32)  [unwired: 1 out]
                n177 = property on="Test Ring" class="Ring (strict)"("Value"=w293, "Strings []"=w292) -> ()  [unwired: 2 in, 2 out]
                n178 = property on="Test Ring" class="Ring (strict)"("Visible"=TRUE) -> ()  [unwired: 2 in, 2 out]
                n179 = property on="Test Slider" class="Slide (strict)"("Visible"=FALSE) -> ()  [unwired: 2 in, 2 out]
              }
              frame "Color Enable  **" {
                n180 = Index Array(array=w304, index=4) -> (element=w305:cluster{string[]})
                n181 = call <vilib>:"NT Read String.vi"("Name"=w307) -> ("String"=w306:string)  [unwired: 9 in, 1 out]
                n182 = Unbundle(w305) -> (w301:string[])
                n183 = Match First String(2:w301, 3:w306) -> (0:w302:i32)  [unwired: 1 out]
                n184 = property on="Test Ring" class="Ring (strict)"("Value"=w302, "Strings []"=w301) -> ()  [unwired: 2 in, 2 out]
                n185 = property on="Test Ring" class="Ring (strict)"("Visible"=TRUE) -> ()  [unwired: 2 in, 2 out]
                n186 = property on="Test Slider" class="Slide (strict)"("Visible"=FALSE) -> ()  [unwired: 2 in, 2 out]
              }
              frame Default {
                n187 = property on="Test Ring" class="Ring (strict)"("Visible"=FALSE) -> ()  [unwired: 2 in, 2 out]
                n188 = property on="Test Slider" class="Slide (strict)"("Visible"=FALSE) -> ()  [unwired: 2 in, 2 out]
              }
              frame "Brightness  **", "Color Level  **", "Compression  **", "FPS  **", "Sharpness  **" {
                n189 = call <vilib>:"NT Read Number.vi"("Name"=w313) -> ("Numeric"=w312:dbl)  [unwired: 9 in, 1 out]
                n190 = local write "Test Slider"(w312) -> ()
                n191 = property on="Test Slider" class="Slide (strict)"("Visible"=TRUE, "Scale.Maximum"=100.0 ("Scale.Range:Maximum")) -> ()  [unwired: 2 in, 2 out]
                n192 = property on="Test Ring" class="Ring (strict)"("Visible"=FALSE) -> ()  [unwired: 2 in, 2 out]
              }
            }
          }
        }
        n193 = property on="Progress" class="Clust (strict)"("Visible"=FALSE) -> ()  [unwired: 2 in, 2 out]
      }
      event "Test Name": Mouse Enter {
        # "Populate the ring with the list of tests"
        n194 = event-data() -> ()  [unwired: 1 in, 1 out]
        n195 = call <vilib>:"NT Read String Array.vi"("Name"="TestMode/TestList") -> ("String Array"=w321:string[])  [unwired: 9 in, 1 out]
        n196 = Build Array (concatenate)("Select the test to run...", w321) -> (w320:string[])
        n197 = property on="Test Name" class="Ring (strict)"("Strings []"=w320) -> ()  [unwired: 2 in, 2 out]
      }
      event "Test Name": Value Change {
        w323 = FALSE ("Visible")
        # "Tell the robot the test name to run"
        n198 = event-data() -> ("NewVal"=w327:u16)  [unwired: 1 in]
        n199 = property on="Test Name" class="Ring (strict)"() -> ("Strings []"=w328:string[])  [unwired: 2 in, 2 out]
        n200 = local write "Progress"(T8 {"Test Progress"=0, "Test Progress Text"=""} ("Progress")) -> ()
        n201 = Index Array(array=w328, index=w327) -> (element=w326:string)
        n202 = call <vilib>:"NT Write String.vi"("String"=w326, "Name"="TestMode/TestName") -> ()  [unwired: 9 in, 1 out]
        n203 = property on="Progress" class="Clust (strict)"("Visible"=TRUE) -> ()  [unwired: 2 in, 2 out]
        n204 = property on="Motor" class="Clust (strict)"("Visible"=w323) -> ()  [unwired: 2 in, 2 out]
        n205 = property on="Test Slider" class="Slide (strict)"("Visible"=w323) -> ()  [unwired: 2 in, 2 out]
        n206 = property on="On/Off" class="Bool (strict)"("Visible"=w323) -> ()  [unwired: 2 in, 2 out]
        n207 = property on="Rev/Fwd" class="Clust (strict)"("Visible"=w323) -> ()  [unwired: 2 in, 2 out]
        n208 = property on="Test Ring" class="Ring (strict)"("Visible"=w323) -> ()  [unwired: 2 in, 2 out]
      }
      event "Listbox": Double Click {
        n209 = event-data() -> ("PlatMods.Shift"=w331:bool, "Row"=w333:i32)  [unwired: 1 in]
        n210 = case shown="True" w331 {
          tunnel: w333 -> [w337 _]
          tunnel: 1 -> [w336 _]
          frame False {
            n211 = property on="Listbox" class="LstBox (strict)"() -> ("Item Symbols"=w335:i32[])  [unwired: 2 in, 2 out]
            n212 = Replace Array Subset(array=w335, new element=w336, index=w337) -> (w334:i32[])
            n213 = property on="Listbox" class="LstBox (strict)"("Item Symbols"=w334) -> ()  [unwired: 2 in, 2 out]
          }
          frame True {
            w338 = 0 ("Top Row")
            n214 = property on="Listbox" class="LstBox (strict)"() -> ("Number of Rows"=w340:u32)  [unwired: 2 in, 2 out]
            n215 = Initialize Array(0, w340) -> (w339:i32[])
            n216 = property on="Listbox" class="LstBox (strict)"("Top Row"=w338, "Value"=w338, "Item Symbols"=w339) -> ()  [unwired: 2 in, 2 out]
          }
        }
      }
      event "Listbox": Key Down {
        n217 = event-data() -> ("VKey"=w344:T16)  [unwired: 1 in]
        n218 = case shown="\"Left\", \"Right\"" w344 {
          selector: w344 -> [w349 _]
          tunnel: eventvkey."Left" ("VKey") -> [w347 _]
          frame "Left", "Right" {
            n219 = Equal?(x=w347, y=w349) -> (x = y?=w348:bool)
            n220 = Select(t=0, s=w348, f=1) -> (s? t:f=w350:i32)
            n221 = property on="Listbox" class="LstBox (strict)"() -> ("Item Symbols"=w353:i32[])  [unwired: 2 in, 2 out]
            n222 = Replace Array Subset(array=w353, new element=w350, index="Listbox") -> (w352:i32[])
            n223 = property on="Listbox" class="LstBox (strict)"("Item Symbols"=w352) -> ()  [unwired: 2 in, 2 out]
          }
          frame Default {
          }
        }
      }
      event "DB Camera Config": Value Change {
        n224 = event-data() -> ("NewVal"=w357:bool)  [unwired: 1 in]
        n225 = case shown="False" w357 {
          tunnel: w356 -> [w366 _]
          tunnel: [w359 w377] -> w355
          tunnel: w354 -> [w358 w377]
          frame False {
            w373 = "Camera"
            w376 = FALSE ("Visible")
            n226 = local read "Camera Settings"() -> (w365:T2)
            n227 = Index Array(array=w366) -> (element=w369:cluster{string[]})  [unwired: 1 in]
            n228 = Unbundle(w365) -> ("Frame Rate"=w364:i32, "Compression"=w363:i32, "Size"=w367:u16)
            n229 = Unbundle(w369) -> (w368:string[])
            n230 = Index Array(array=w368, index=w367) -> (element=w362:string)
            n231 = call-poly <vilib>:"Write Key.vi"("section"=w373, "value"=w362, "key"="Size", "refnum"=w358) -> ("refnum out"=w375:T15)  [unwired: 2 in, 5 out]
            n232 = call-poly <vilib>:"Write Key.vi"("section"=w373, "value"=w364, "key"="FrameRate", "refnum"=w375) -> ("refnum out"=w374:T15)  [unwired: 1 in, 6 out]
            n233 = property on="Camera Settings" class="Clust (strict)"("Visible"=w376) -> ()  [unwired: 2 in, 2 out]
            n234 = local write "DB Camera Config"(w376) -> ()
            n235 = call-poly <vilib>:"Write Key.vi"("section"=w373, "value"=w363, "key"="Compression", "refnum"=w374) -> ("refnum out"=w360:T15)  [unwired: 1 in, 6 out]
            n236 = call <vilib>:"Close Config Data.vi"("refnum"=w360) -> ("file path"=w361:path)  [unwired: 2 in, 8 out]
            n237 = call <vilib>:"Open Config Data.vi"("configuration file path"=w361) -> ("refnum"=w359:T15)  [unwired: 8 in, 2 out]
          }
          frame True {
            n238 = property on="Camera Settings" class="Clust (strict)"("Visible"=TRUE) -> ()  [unwired: 2 in, 2 out]
          }
        }
      }
      event "Camera Settings": Value Change {
        n239 = event-data() -> ("NewVal"=w390:T2)  [unwired: 1 in]
        n240 = Index Array(array=w386) -> (element=w385:cluster{string[]})  [unwired: 1 in]
        n241 = Unbundle(w390) -> ("Frame Rate"=w381:i32, "Compression"=w380:i32, "Size"=w383:u16)
        n242 = Unbundle(w385) -> (w384:string[])
        n243 = Index Array(array=w384, index=w383) -> (element=w382:string)
        n244 = Format Into String(format string="%s   %dfps   %d%%", w382, w381, w380) -> (resulting string=w387:string)  [unwired: 2 in, 1 out]
        n245 = Build Array(w387) -> (w388:string[])
        n246 = property on="DB Camera Config" class="Bool (strict)"("Strings [4]"=w388) -> ()  [unwired: 2 in, 2 out]
      }
      event "Motor.Enable": Value Change {
        n247 = event-data() -> ("NewVal"=w396:bool)  [unwired: 1 in]
        n248 = Unbundle("Motor") -> ("Value"=w395:dbl)  [unwired: 1 out]
        n249 = Select(t=w395, s=w396, f=0.0) -> (s? t:f=w393:dbl)
        n250 = call <vilib>:"NT Write Number.vi"("Numeric"=w393, "Name"=w392) -> ()  [unwired: 9 in, 1 out]
      }
      event "Test Slider": Value Change {
        n251 = event-data() -> ("NewVal"=w399:dbl)  [unwired: 1 in]
        n252 = call <vilib>:"NT Write Number.vi"("Numeric"=w399, "Name"=w400) -> ()  [unwired: 9 in, 1 out]
      }
      event "On/Off": Value Change {
        n253 = event-data() -> ("NewVal"=w404:bool)  [unwired: 1 in]
        n254 = Boolean To (0,1)(Boolean=w404) -> (0, 1=w403:i16)
        n255 = call <vilib>:"NT Write Number.vi"("Numeric"=w403, "Name"=w402) -> ()  [unwired: 9 in, 1 out]
      }
      event "Rev/Fwd": Value Change {
        n256 = event-data() -> ("NewVal.Forward"=w412:bool, "NewVal.Reverse"=w411:bool)  [unwired: 1 in]
        n257 = Boolean To (0,1)(Boolean=w412) -> (0, 1=w408:i16)
        n258 = Boolean To (0,1)(Boolean=w411) -> (0, 1=w410:i16)
        n259 = Negate(x=w410) -> (-x=w409:i16)
        n260 = Add(x=w408, y=w409) -> (x+y=w407:i16)
        n261 = call <vilib>:"NT Write Number.vi"("Numeric"=w407, "Name"=w406) -> ()  [unwired: 9 in, 1 out]
      }
      event "Test Ring": Value Change {
        n262 = event-data() -> ("NewVal"=w416:u16)  [unwired: 1 in]
        n263 = property on="Test Ring" class="Ring (strict)"() -> ("Strings []"=w417:string[])  [unwired: 2 in, 2 out]
        n264 = Index Array(array=w417, index=w416) -> (element=w415:string)
        n265 = call <vilib>:"NT Write String.vi"("String"=w415, "Name"=w414) -> ()  [unwired: 9 in, 1 out]
      }
      event "Rec Mode": Value Change {
        # "Update globals for recording mode and path to read log from.\nClear when logging and let NetworkTables set path for vision to\nuse."
        n266 = event-data() -> ("NewVal"=w427:enum32{"Stop", "Record", "Playback"})  [unwired: 1 in]
        n267 = global write "WPI_DashboardLogging Global.vi" "Logging Filename"(path "") -> ()
        n268 = case shown="\"Stop\", \"Record\"" w427 {
          tunnel: w426 -> [_ w429 w437]
          tunnel: [_ _ w436] -> w423
          tunnel: [_ _ w435] -> _
          tunnel: w421 -> [_ _ w433]
          tunnel: cluster{i32, i32} {-250, 170} -> [_ _ w432]
          tunnel: [_ _ T17 {"Image Size"=TRUE, "Image Type"=TRUE, "Pixel Value"=TRUE, "ROI Information"=TRUE, "Zoom Factor"=FALSE} ("Image Information Shown:All Elements")] -> w419
          tunnel: [_ _ TRUE ("Zoom Factor")] -> w418
          frame Default {
          }
          frame "Stop", "Record" {
            # "Place Window too"
            n269 = invoke class="VI" method="FP.Close"(reference=w429) -> (reference out=w428:refnum<vi>)  [unwired: 2 in, 2 out]
            n270 = invoke class="VI" method="Abort VI"(reference=w428) -> ()  [unwired: 2 in, 3 out]
          }
          frame "Playback" {
            n271 = call "Open Playback Panel.vi"("Offset"=w432, "DB VI Ref"=w433, "Playback in"=w437) -> ("Playback out"=w434:refnum<vi>)  [unwired: 8 in]
            n272 = register-events(w434) -> (reference out=w436:refnum<event-registration>, error out=w435:errorcluster)  [unwired: 2 in]
          }
        }
        n273 = global write "WPI_DashboardLogging Global.vi" "Recording"(w427) -> ()
        n274 = property on="Camera Image" class="ImageControl"("Image Information Shown"=w419, "Image Information Visible"=w418) -> ()  [unwired: 2 in, 2 out]
        n275 = call <vilib>:"WPI_DashboardNT Log FieldName Cache.vi"("Operation"=enum16{"Lookup/Add", "Index", "Clear"}."Clear") -> ()  [unwired: 8 in, 3 out]
      }
      event Panel Close {
        w438 = enum32{"Stop", "Record", "Playback"}."Stop" ("Rec Mode")
        n276 = event-data() -> ()  [unwired: 1 in, 4 out]
        n277 = local write "Rec Mode"(w438) -> ()
        n278 = global write "WPI_DashboardLogging Global.vi" "Recording"(w438) -> ()
      }
      event Panel Close {
        # "Abort playback window and ourself"
        n279 = event-data() -> ()  [unwired: 1 in, 4 out]
        n280 = invoke class="VI" method="FP.Close"(reference=w443) -> (reference out=w442:refnum<vi>)  [unwired: 2 in, 2 out]
        n281 = invoke class="VI" method="Abort VI"(reference=w442) -> (error out=w441:errorcluster)  [unwired: 2 in, 2 out]
        n282 = invoke class="VI" method="Abort VI"(error in=w441) -> ()  [unwired: 2 in, 3 out]
      }
    }
  }
  n283 = property on="On/Off" class="Bool (strict)"("Visible"=w25) -> ()  [unwired: 2 in, 2 out]
  n284 = property on="Motor" class="Clust (strict)"("Visible"=w25) -> ()  [unwired: 2 in, 2 out]
  n285 = property on="Progress" class="Clust (strict)"("Visible"=w25) -> ()  [unwired: 2 in, 2 out]
  n286 = property on="Test Ring" class="Ring (strict)"("Visible"=w25) -> ()  [unwired: 2 in, 2 out]
  n287 = property on="Rev/Fwd" class="Clust (strict)"("Visible"=w25) -> ()  [unwired: 2 in, 2 out]
  n288 = property on="Camera Settings" class="Clust (strict)"("Visible"=w25) -> ()  [unwired: 2 in, 2 out]
  n289 = local write "DB Camera Config"(w25) -> ()
  n290 = global write "WPI_DashboardLogging Global.vi" "Recording"(w8) -> ()
  n291 = local write "Rec Mode"(w8) -> ()
